vi "Reset.vi"(7 "Address":u16, 8 "Error In":errorcluster, 11 "VISA Resource in":refnum<visa-resource-name>) -> (0 "Error Out":errorcluster, 3 "VISA Resource out":refnum<visa-resource-name>)   [LabVIEW 2015, in "KIT QV.lvlib"]
doc: "Resets the instrument, wait 10 s after, and then sends a set of default setup commands to the instrument."
uses:
  KIT QV.lvlib
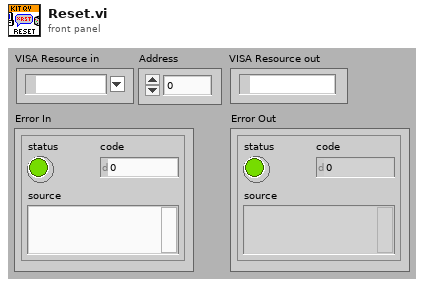
[diagram p1: front panel]
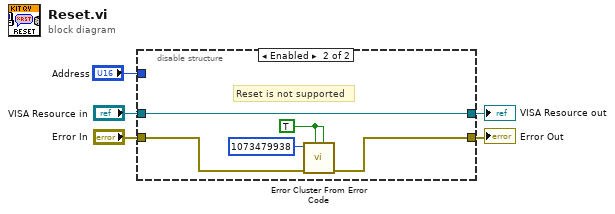
[diagram p0: block diagram]
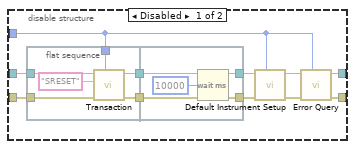
[diagram p2: hidden frame]
diagram:
  n1 = disable-structure shown="Enabled" {
    disable-tunnel: [w12 w30] -> w5
    disable-tunnel: [w11 w27] -> w4
    disable-tunnel: "VISA Resource in" -> [w10 w30]
    disable-tunnel: "Error In" -> [w7 w28]
    disable-tunnel: "Address" -> [w6 _]
    frame Disabled {
      n2 = flat-sequence {
        tunnel: w10 -> [w22]
        tunnel: w7 -> [w19]
        tunnel: w6 -> [w18]
        tunnel: [w21] -> w16
        tunnel: [w20] -> w15
        tunnel: [w24] -> w8
        tunnel: [w25] -> w9
        tunnel: w16 -> [w25]
        tunnel: w15 -> [w24]
        frame #0 {
          n3 = call "Transaction.vi"("Address"=w18, "error in (no error)"=w19, "Command"="SRESET" ("Reset Command"), "VISA Resource in"=w22) -> ("error out"=w20:errorcluster, "VISA Resource out"=w21:refnum<visa-resource-name>)  [unwired: 5 in, 1 out]
        }
        frame #1 {
          n4 = Wait (ms)(milliseconds to wait=u32 10000) -> ()  [unwired: 1 out]
        }
      }
      n5 = call "Default Instrument Setup.vi"("Address"=w6, "Error In"=w8, "VISA Resource in"=w9) -> ("Error Out"=w14:errorcluster, "VISA Resource out"=w13:refnum<visa-resource-name>)  [unwired: 7 in]
      n6 = call "Error Query.vi"("Address"=w6, "Error in"=w14, "VISA Resource in"=w13) -> ("Error Out"=w11:errorcluster, "VISA Resource in"=w12:refnum<visa-resource-name>)  [unwired: 5 in, 2 out]
    }
    frame Enabled {
      w26 = TRUE ("show call chain? (False)")
      # "Reset is not supported"
      n7 = call <vilib>:"Error Cluster From Error Code.vi"("is warning? (False)"=w26, "show call chain? (False)"=w26, "error in (no error)"=w28, "error code (0)"=1073479938) -> ("error out"=w27:errorcluster)  [unwired: 5 in]
    }
  }
  "Error Out" <- w4
  "VISA Resource out" <- w5
